vi "Read Test Type.vi"(11 "Test in":refnum<class "Test.lvclass">) -> (2 "Test Type":string)   [LabVIEW 2018, in "Test.lvclass"]
uses:
  Test.lvclass
  Test.lvclass/Test.ctl
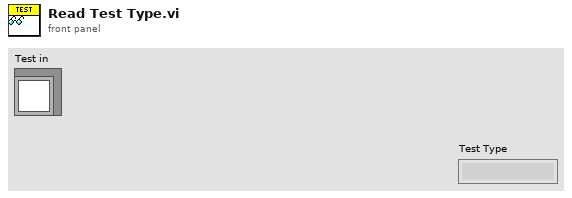
[diagram p1: front panel]
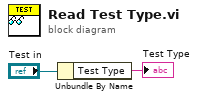
[diagram p0: block diagram]
diagram:
  n1 = Unbundle By Name("Test in") -> ("Test Type"=→"Test Type":string)
